vi "ModeLED.vi"(9 "Locate LED":bool, 10 "Choose Hue":bool) -> (2 "LED Mode":T1(ring))   [LabVIEW 2020]
doc: "Determines the appropriate LED mode based on the robot state, driver inputs, and live deploy configuration."
uses:
  driverdata.vi
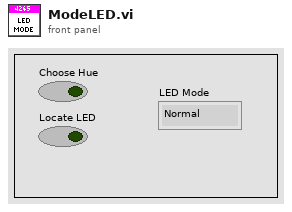
[diagram p1: front panel]
types:
  T1 = enum16{"Normal", "Party Mode", "Choose Hue", "Debug", "Locate LED", "Distance Rainbow"}
  T2 = enum16{"Center", "North", "NorthWest", "West", "SouthWest", "South", "SouthEast", "East", "NorthEast"}
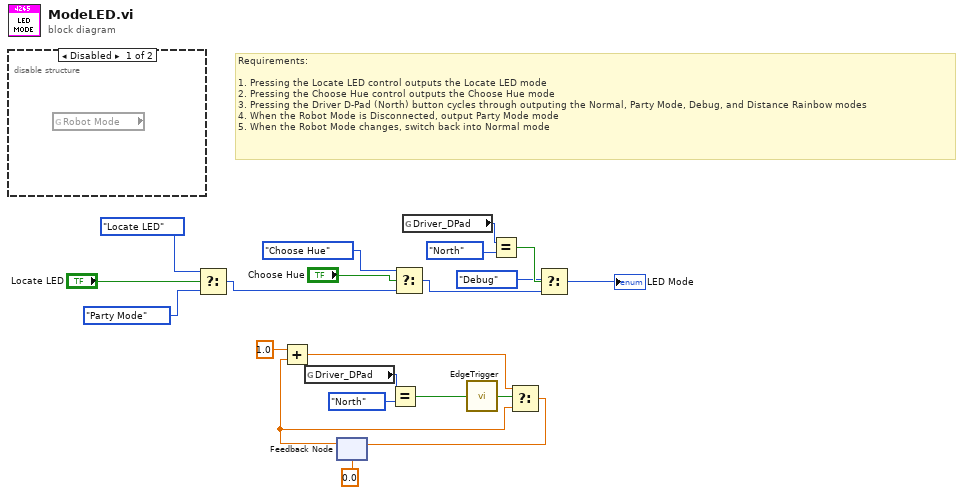
[diagram p0: block diagram]
diagram:
  # "Requirements:\n\n1. Pressing the Locate LED control outputs the Locate LED mode\n2. Pressing the Choose Hue control outputs the Choose Hue mode\n3. Pressing the Driver D-Pad (North) button cycles through outputing the Normal, Party Mode, Debug, and Distance Rainbow modes\n4. When the Robot Mode is Disconnected, output Party Mode mode\n5. When the Robot Mode changes, switch back into Normal mode"
  n1 = disable-structure shown="Disabled" {
    frame Disabled {
      n2 = global read "driverdata.vi" "Robot Mode"() -> ()  [unwired: 1 out]
    }
    frame Enabled {
    }
  }
  n3 = Select(t=T1."Locate LED", s="Locate LED", f=T1."Party Mode") -> (s? t:f=w17:T1)
  n4 = global read "driverdata.vi" "Driver_DPad"() -> (w3:T2)
  n5 = feedback #1(0.0) -> (w5:dbl)
  n6 = Add(x=1.0, y=w5) -> (x+y=w7:dbl)
  n7 = Equal?(x=w3, y=T2."North" ("Driver_DPad")) -> (x = y?=w2:bool)
  n8 = Select(t=T1."Choose Hue", s="Choose Hue", f=w17) -> (s? t:f=w11:T1)
  n9 = global read "driverdata.vi" "Driver_DPad"() -> (w14:T2)
  n10 = call "EdgeTrigger.vi"("Input Signal"=w2) -> ("All Edge Trigger"=w1:bool)  [unwired: 2 out]
  n11 = Equal?(x=w14, y=T2."North" ("Driver_DPad")) -> (x = y?=w13:bool)
  n12 = Select(t=w7, s=w1, f=w5) -> (s? t:f=w6:dbl)
  n13 = feedback-in #1(w6) -> ()
  n14 = Select(t=T1."Debug", s=w13, f=w11) -> (s? t:f=→"LED Mode":T1)
